vi "Get Data.vi"(8 "error in (no error)":errorcluster, 11 "TriggerAction in":refnum<class "TriggerAction Q.lvclass">) -> (0 "error out":errorcluster, 2 "Array of TriggerAction Elements":T1[](array[typedef]), 3 "TriggerAction out":refnum<class "TriggerAction Q.lvclass">)   [LabVIEW 2016, in "TriggerAction Q.lvclass"]
uses:
  <userlib>/Common Components/TriggerAction Q/TriggerAction Q/TriggerAction Q.lvclass
  <userlib>/Common Components/TriggerAction Q/TriggerAction Q/Element Data.ctl
  <userlib>/Common Components/TriggerAction Q/TriggerAction Q/TriggerAction Q.lvclass/TriggerAction Q.ctl
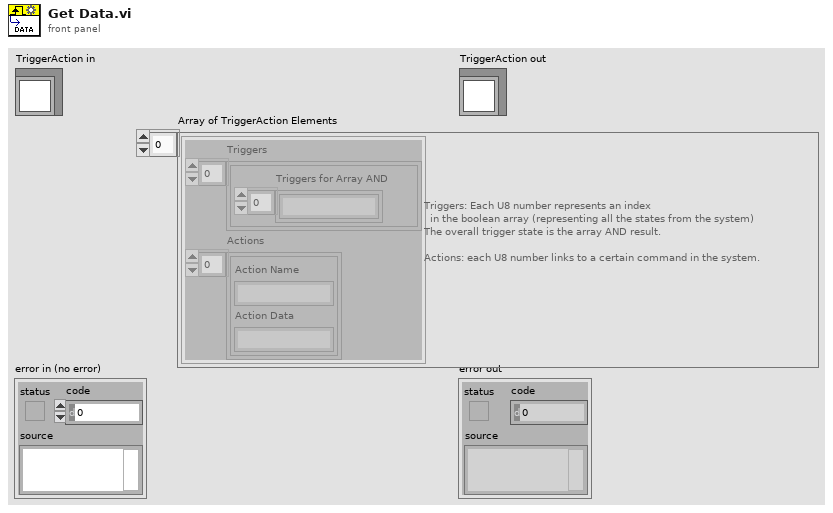
[diagram p1: front panel]
types:
  T1 = typedef "TriggerAction Q.lvclass/Element Data.ctl" = cluster{"Triggers":cluster{"Triggers for Array AND":string[]}[], "Actions":cluster{"Action Name":string, "Action Data":string}[]}
  T2 = typedef "TriggerAction.lvclass/Element Data.ctl" = cluster{"Triggers":cluster{"Triggers for Array AND":string[]}[], "Actions":cluster{"Action Name":string, "Action Data":string}[]}
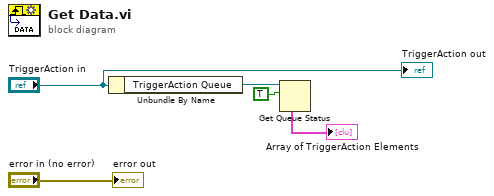
[diagram p0: block diagram]
diagram:
  n1 = Unbundle By Name("TriggerAction in") -> ("TriggerAction Queue"=w3:refnum<queue>)
  n2 = Get Queue Status(queue=w3, return elements? (F)=TRUE) -> (elements=→"Array of TriggerAction Elements":T2[])  [unwired: 1 in, 7 out]
  "error out" <- "error in (no error)"
  "TriggerAction out" <- "TriggerAction in"
